vi "update_data_representation_partSD.vi"(0 "Item Names":string[](array[string]), 1 "Commentaires exp":refnum<vi>, 2 "# exp":i32, 3 "Experiment":T1, 4 "error in (no error)":errorcluster, 5 "Experiments group":refnum<class "Experiments_group.lvclass">[](array[class]), 7 "Group":u16) -> (6 "timedelays":dbl[](array[numeric]), 8 "error out":errorcluster, 9 "wavelengths":dbl[](array[numeric]), 10 "Data":dbl[][](array[numeric]))   [LabVIEW 2015]
uses:
  Classes/Experiments_group.lvclass
  controls/mylistboxRef.ctl
  controls/mylistbox.ctl
  Classes/Experiment.lvclass
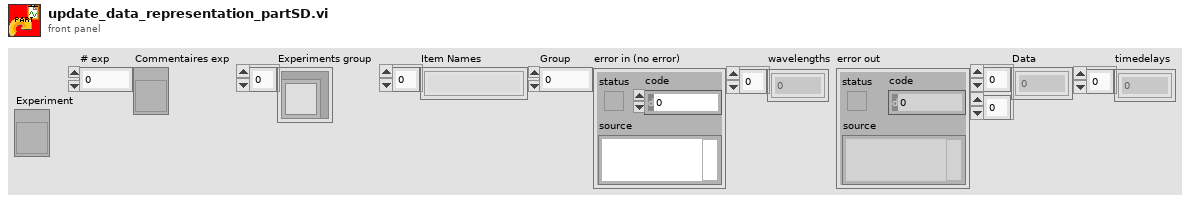
[diagram p1: front panel]
types:
  T1 = typedef "mylistboxRef.ctl" = refnum<vi>
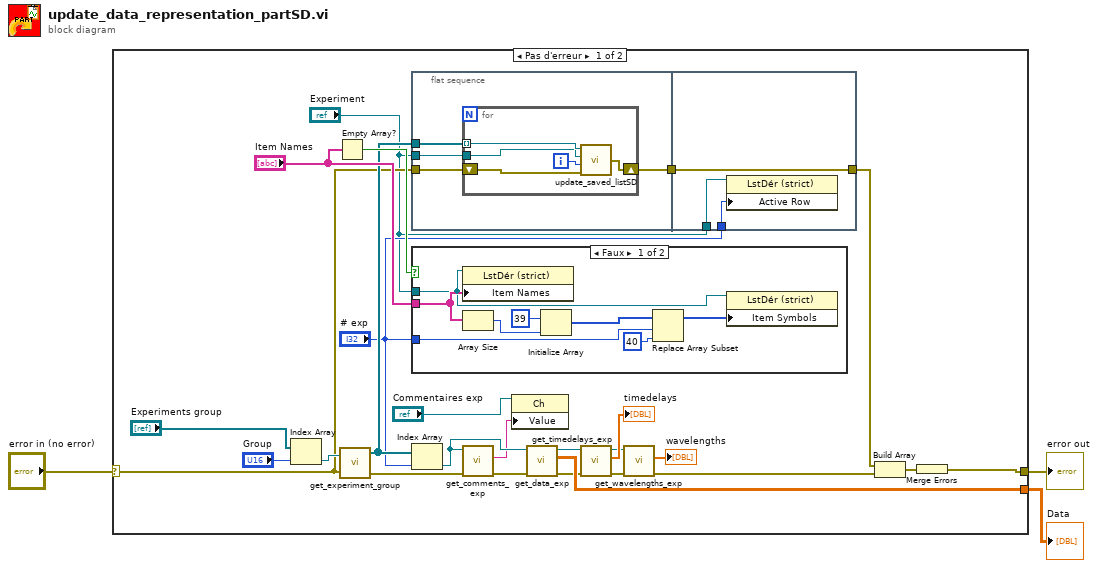
[diagram p0: block diagram]
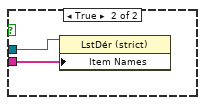
[diagram p2: hidden frame]
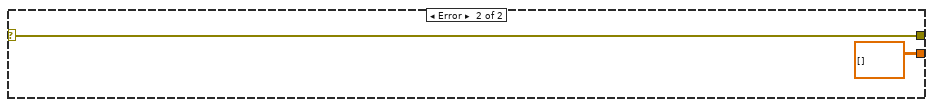
[diagram p3: hidden frame]
diagram:
  n1 = case shown="Pas d'erreur" "error in (no error)" {
    selector: "error in (no error)" -> [w16 w53]
    tunnel: [w17 w53] -> w2
    tunnel: [w22 dbl[][] [] ("Data")] -> w1
    frame No Error {
      n2 = Index Array(array="Experiments group", index="Group") -> (element=w24:refnum<class "Experiments_group.lvclass">)
      n3 = Empty Array?(array="Item Names") -> (empty?=w29:bool)
      n4 = call-dynamic "get_experiment_group.vi"("Experiments_group.lvclass in"=w24, "error in (no error)"=w16) -> ("Experiments"=w19:refnum<class "Experiment.lvclass">[], "error out"=w10:errorcluster)  [unwired: 1 out]
      n5 = flat-sequence {
        tunnel: "Experiment" -> [w33]
        tunnel: w19 -> [w32]
        tunnel: w16 -> [w30]
        tunnel: [w31] -> w15
        tunnel: [w41] -> w18
        tunnel: w15 -> [w41]
        tunnel: "Experiment" -> [w40]
        tunnel: "# exp" -> [w39]
        frame #0 {
          n6 = for {
            tunnel: w33 -> [w34]
            tunnel: w32 -> [w38] mode=indexing
            shift-right: [w36] -> w31
            shift-left: w30 -> [w35]
            i -> [w37]
            n7 = call "update_saved_listSD.vi"("error in (no error)"=w35, "Numeric"=w37, "Experiment"=w34, "Experiment in"=w38) -> ("error out"=w36:errorcluster)
          }
        }
        frame #1 {
          n8 = property on="Property Node" class="LstDér (strict)"(reference=w40, "Active Row"=w39) -> ()  [unwired: 1 in, 2 out]
        }
      }
      n9 = case shown="Faux" w29 {
        tunnel: "Item Names" -> [w44 w51]
        tunnel: "Experiment" -> [w43 w50]
        tunnel: "# exp" -> [w42 _]
        frame False {
          n10 = property on="Property Node" class="LstDér (strict)"(reference=w43, "Item Names"=w44) -> ()  [unwired: 1 in, 2 out]
          n11 = Array Size(array=w44) -> (size(s)=w45:i32)
          n12 = Initialize Array(39, w45) -> (w47:i32[])
          n13 = Replace Array Subset(array=w47, new element=40 ("new element/subarray"), index=w42) -> (w46:i32[])
          n14 = property on="Property Node" class="LstDér (strict)"(reference=w43, "Item Symbols"=w46) -> ()  [unwired: 1 in, 2 out]
        }
        frame True {
          n15 = property on="Property Node" class="LstDér (strict)"(reference=w50, "Item Names"=w51) -> ()  [unwired: 1 in, 2 out]
        }
      }
      n16 = Index Array(array=w19, index="# exp") -> (element=w27:refnum<class "Experiment.lvclass">)
      n17 = call-dynamic "get_comments_exp.vi"("error in (no error)"=w10, "Experiment.lvclass in"=w27) -> ("error out"=w23:errorcluster, "Comments"=w25:string)  [unwired: 7 in, 1 out]
      n18 = property class="Ch"(reference="Commentaires exp", "Value"=w25) -> ()  [unwired: 1 in, 2 out]
      n19 = call-dynamic "get_data_exp.vi"("error in (no error)"=w23, "Experiment.lvclass in"=w27) -> ("error out"=w11:errorcluster, "Data"=w22:dbl[][], "Experiment.lvclass out"=w13:refnum<class "Experiment.lvclass">)  [unwired: 7 in]
      n20 = call-dynamic "get_timedelays_exp.vi"("error in (no error)"=w11, "Experiment.lvclass in"=w13) -> ("error out"=w8:errorcluster, "timedelays"=→"timedelays":dbl[], "Experiment.lvclass out"=w9:refnum<class "Experiment.lvclass">)  [unwired: 7 in]
      n21 = call-dynamic "get_wavelengths_exp.vi"("error in (no error)"=w8, "Experiment.lvclass in"=w9) -> ("error out"=w7:errorcluster, "wavelengths"=→"wavelengths":dbl[])  [unwired: 7 in, 1 out]
      n22 = Build Array(w18, w7) -> (w5:errorcluster[])
      n23 = Merge Errors(w5) -> (w17:errorcluster)
    }
    frame Error {
    }
  }
  "error out" <- w2
  "Data" <- w1
